vi "Control_ReadJoystick.vi"(1 "joy_left [FPGA DI]":refnum<k21>="ConnectorA/DIO0", 4 "joy_right [FPGA DI]":refnum<k21>="ConnectorA/DIO0") -> (15 "Left":bool, 18 "Right":bool)   [LabVIEW 2018]
uses:
  <vilib>/rvi/eio/common/nirviEmuTemplateMethod_errors.vi
  <vilib>/eio/EIONode/EIONode.xnode
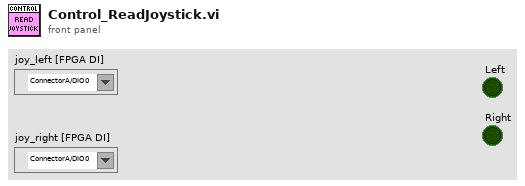
[diagram p1: front panel]
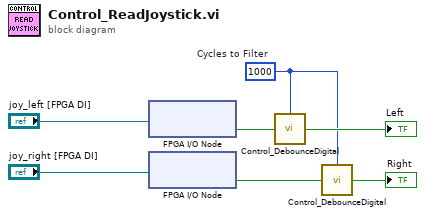
[diagram p0: block diagram]
diagram:
  w5 = u16 1000  # Cycles to Filter
  n1 = xnode "FPGA I/O Node"("FPGA I/O In"="joy_left [FPGA DI]") -> ("I/O Item"=w3:bool)  [unwired: 1 out]
  n2 = xnode "FPGA I/O Node"("FPGA I/O In"="joy_right [FPGA DI]") -> ("I/O Item"=w1:bool)  [unwired: 1 out]
  n3 = call "Control_DebounceDigital.vi"("Input Signal"=w3, "Cycles to Filter"=w5) -> ("Output Filtered Signal"=→"Left":bool)
  n4 = call "Control_DebounceDigital.vi"("Input Signal"=w1, "Cycles to Filter"=w5) -> ("Output Filtered Signal"=→"Right":bool)
